vi "DHE_DO_IMREAD.vi"(8 "error in":errorcluster) -> (0 "error out":errorcluster, 2 "response":string)   [LabVIEW 2016]
uses:
  SDSU_GBLVariables.vi
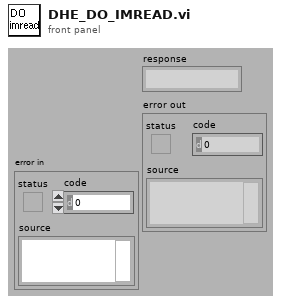
[diagram p1: front panel]
types:
  T1 = typedef "DatabaseHand_RefNum.ctl" = refnum<vi>
  T2 = typedef "CMN_TimingInfo.ctl" = cluster{"PixelTime":sgl, "SkipPixel":sgl, "SkipRow":sgl, "ShiftRow":sgl, "ShiftedPix":u16, "known_overhead":sgl, "DET_READ_TIME":sgl}
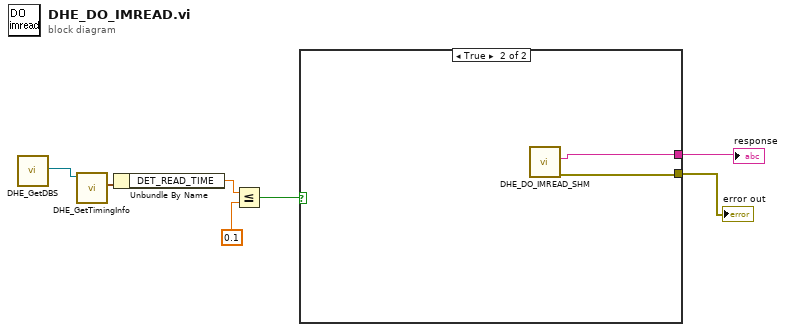
[diagram p0: block diagram]
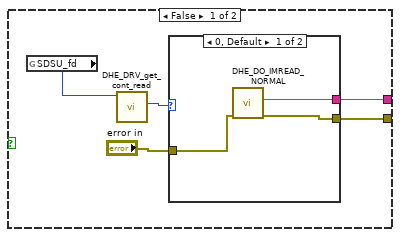
[diagram p2: hidden frame]
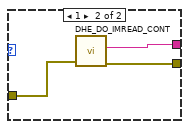
[diagram p3: hidden frame]
diagram:
  n1 = call "DHE_GetDBS.vi"() -> ("DHE_DBSRef"=w3:T1)  [unwired: 9 out]
  n2 = call "DHE_GetTimingInfo.vi"("Database RefNum out"=w3) -> ("Timing"=w2:T2)  [unwired: 10 out]
  n3 = Unbundle By Name(w2) -> ("DET_READ_TIME"=w1:sgl)
  n4 = Less Or Equal?(x=w1, y=0.1) -> (x <= y?=w4:bool)
  n5 = case shown="True" w4 {
    tunnel: [w9 w19] -> w7
    tunnel: [w8 w20] -> w6
    frame False {
      n6 = global read "SDSU_GBLVariables.vi" "SDSU_fd"() -> (w12:i32)
      n7 = call "DHE_DRV_get_cont_read.vi"("fd"=w12) -> ("cont_read"=w11:i32)  [unwired: 1 in, 9 out]
      n8 = case shown="0, Default" w11 {
        tunnel: "error in" -> [w15 w18]
        tunnel: [w14 w17] -> w9
        tunnel: [w13 w16] -> w8
        frame 0, Default {
          n9 = call "DHE_DO_IMREAD_NORMAL.vi"("error in"=w15) -> ("error out"=w13:errorcluster, "response"=w14:string)  [unwired: 9 out]
        }
        frame 1 {
          n10 = call "DHE_DO_IMREAD_CONT.vi"("error in"=w18) -> ("error out"=w16:errorcluster, "response"=w17:string)  [unwired: 9 out]
        }
      }
    }
    frame True {
      n11 = call "DHE_DO_IMREAD_SHM.vi"() -> ("error out"=w20:errorcluster, "response"=w19:string)  [unwired: 1 in, 9 out]
    }
  }
  "response" <- w7
  "error out" <- w6
